vi "Process Records.vi"(4 "map from message info to indexes":T1, 5 "RT hardware channel data":T2[](array[typedef])=[{"channel #"=0, "channel handle"=0, "labels settings for RT"=[]}] {"labels settings for RT"."Label Timestamp Channel Data Reference" format="%.0x"; "labels settings for RT"."Word Initial Raw Value" format="%032.0f"; "labels settings for RT"."Label Disable/Trigger Channel Reference" format="%.0x"; "labels settings for RT"."parameter driver data"."Tx parameter refs" format="%.0x"; "labels settings for RT"."SDI" format="%02b"; "labels settings for RT"."label" format="%.0o"}, 6 "error in":errorcluster, 8 "map from message info to data word":T11(c390), 9 "parameter values in":dbl[](array[numeric])) -> (0 "error out":errorcluster, 3 "parameter values out":dbl[](array[numeric]))   [LabVIEW 2020, in "AIM ARINC 429 Engine.lvlib" / "Custom Device.lvlib"]
uses:
  Custom Device.lvlib
  ece6b673-d70a-4abd-8fc5-cd5ecd079ce2.vi
  <vilib>/NI VeriStand/Custom Device API/Data Reference.ctl
  <vilib>/NI VeriStand/Custom Device API/Custom Device API.lvlib
  <vilib>/NI VeriStand/Custom Device API/Custom Device Item Ref.ctl
  Shared/Label.ctl
  <vilib>/NI/NI VeriStand Encoding and Decoding/Encoding.ctl
  <vilib>/NI/NI VeriStand Encoding and Decoding/Encoding and Decoding.lvlib
  Shared/Parameter Definition.ctl
  Shared/RT Parameters.ctl
  Shared/Transfer Type.ctl
  Shared/RT Label Settings.ctl
  Shared/RT Hardware Channel Settings.ctl
  Shared/Map of Identifiers to Indexes.ctl
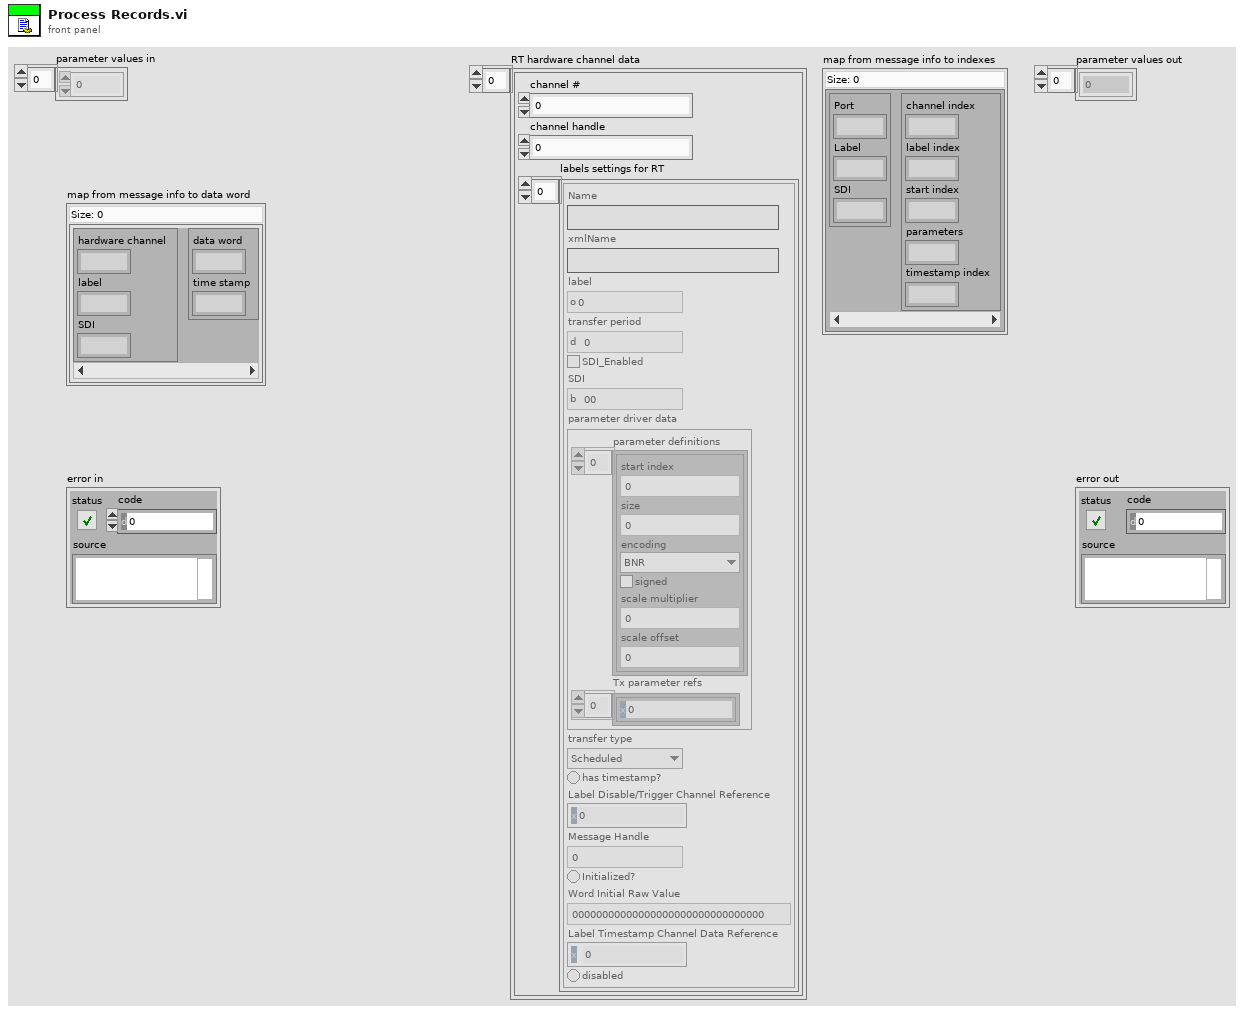
[diagram p1: front panel]
types:
  T1 = typedef "Map of Identifiers to Indexes.ctl" = map{cluster{"Port":u8, "Label":u8, "SDI":u8}, cluster{"channel index":i32, "label index":i32, "start index":i32, "parameters":i32, "timestamp index":i32}}
  T2 = typedef "RT Hardware Channel Settings.ctl" = cluster{"channel #":u16, "channel handle":u64, "labels settings for RT":T3[]}
  T3 = typedef "RT Label Settings.ctl" = cluster{"Name":string, "xmlName":string, "label":T4, "transfer period":u32, "SDI_Enabled":bool, "SDI":u8, "parameter driver data":T5, "transfer type":T9, "has timestamp?":bool, "Label Disable/Trigger Channel Reference":T8, "Message Handle":u64, "Initialized?":bool, "Word Initial Raw Value":u32, "Label Timestamp Channel Data Reference":T10, "disabled":bool}
  T4 = typedef "Label.ctl" = u8
  T5 = typedef "RT Parameters.ctl" = cluster{"parameter definitions":T6[], "Tx parameter refs":T8[]}
  T6 = typedef "Parameter Definition.ctl" = cluster{"start index":i32, "size":i32, "encoding":T7, "signed":bool, "scale multiplier":dbl, "scale offset":dbl}
  T7 = typedef "Encoding and Decoding.lvlib/Encoding.ctl" = enum16{"BNR", "BCD", "Discrete"}
  T8 = typedef "Custom Device API.lvlib/Custom Device Item Ref.ctl" = u64
  T9 = typedef "Transfer Type.ctl" = enum16{"Scheduled", "Acyclic", "Block", "Strobe"}
  T10 = typedef "Custom Device API.lvlib/Data Reference.ctl" = i32
  T11 = map{cluster{"hardware channel":u8, "label":u8, "SDI":u8}, cluster{"data word":u32, "time stamp":dbl}}
  T12 = cluster{"hardware channel":u8, "label":u8, "SDI":u8}
  T13 = cluster{"channel index":i32, "label index":i32, "start index":i32, "parameters":i32, "timestamp":i32}
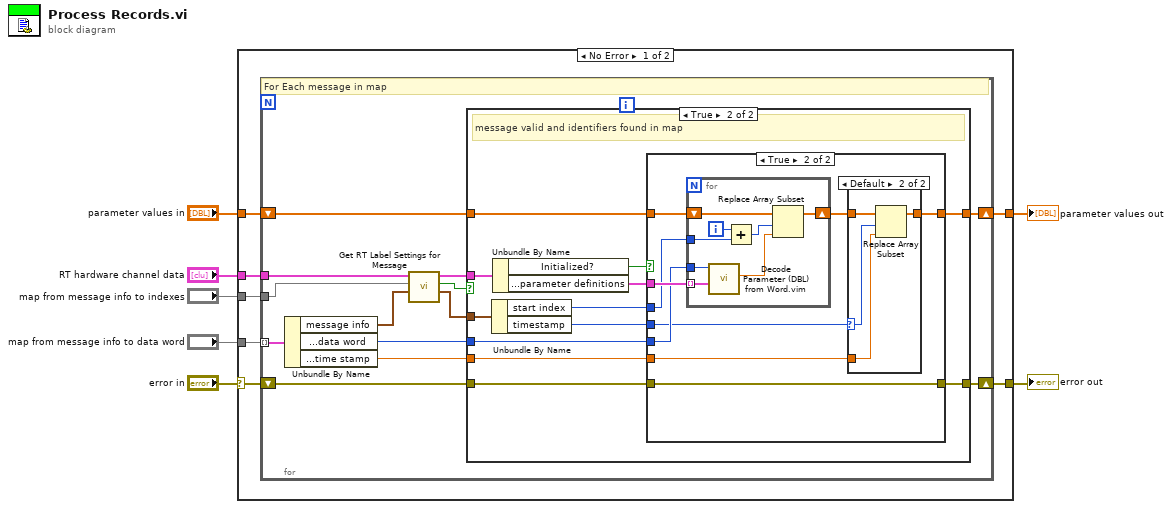
[diagram p0: block diagram]
diagram:
  n1 = case shown="No Error" "error in" {
    selector: "error in" -> [w12 w67]
    tunnel: "map from message info to data word" -> [w11 _]
    tunnel: [w14 w67] -> w6
    tunnel: "RT hardware channel data" -> [w13 _]
    tunnel: [w9 w66] -> w3
    tunnel: "parameter values in" -> [w10 w66]
    tunnel: "map from message info to indexes" -> [w8 _]
    frame No Error {
      n2 = for "Process each Record" {
        tunnel: w11 -> [w16] mode=indexing
        shift-right: [w27] -> w14
        shift-left: w12 -> [w26]
        tunnel: w13 -> [w23]
        shift-right: [w24] -> w9
        shift-left: w10 -> [w25]
        tunnel: w8 -> [w21]
        # "For Each message in map"
        n3 = Unbundle By Name(w16) -> ("message info"=w18:T12, "data word and time stamp.data word"=w17:u32, "data word and time stamp.time stamp"=w15:dbl)
        n4 = call "Get RT Label Settings for Message.vi"("message identifiers"=w18, "map"=w21, "RT hardware channel data"=w23) -> ("message indexes"=w19:T13, "valid and map exists"=w20:bool, "label settings for RT"=w22:T3)  [unwired: 6 in]
        n5 = case "Channel Found?" shown="True" w20 {
          tunnel: w26 -> [w29 w40]
          tunnel: [w29 w39] -> w27
          tunnel: w17 -> [_ w35]
          tunnel: [w28 w38] -> w24
          tunnel: w25 -> [w28 w36]
          tunnel: w22 -> [_ w34]
          tunnel: w19 -> [_ w33]
          tunnel: w15 -> [_ w31]
          frame False {
            # "message not valid or not found in map"
          }
          frame True {
            # "message valid and identifiers found in map"
            n6 = Unbundle By Name(w33) -> ("start index"=w32:i32, "timestamp"=w30:i32)
            n7 = Unbundle By Name(w34) -> ("Initialized?"=w37:bool, "parameter driver data.parameter definitions"=w41:T6[])
            n8 = case shown="True" w37 {
              tunnel: w41 -> [_ w51]
              tunnel: w35 -> [_ w50]
              tunnel: w40 -> [w43 w52]
              tunnel: [w43 w52] -> w39
              tunnel: [w42 w46] -> w38
              tunnel: w36 -> [w42 w49]
              tunnel: w32 -> [_ w48]
              tunnel: w31 -> [_ w44]
              tunnel: w30 -> [_ w47]
              frame False {
                # "This case will be called if users has Labels present on the channel but didn't list them in XML file with \"monitor=false\" in the list.\n\nRecords returned by Read function will have labels (not filtered by HW)."
              }
              frame True {
                n9 = for {
                  tunnel: w51 -> [w65] mode=indexing
                  tunnel: w50 -> [w64]
                  tunnel: w48 -> [w59]
                  shift-right: [w61] -> w45
                  shift-left: w49 -> [w63]
                  i -> [w60]
                  n10 = call "Decode Parameter (DBL) from Word.vim"("parameter definition"=w65, "32-bit word in"=w64) -> ("parameter value"=w62:dbl)  [unwired: 7 in, 2 out]
                  n11 = Add(x=w60, y=w59) -> (x+y=w58:i32)
                  n12 = Replace Array Subset(array=w63, new element=w62, index=w58) -> (w61:dbl[])
                }
                n13 = case shown="Default" w47 {
                  selector: w47 -> [_ w55]
                  tunnel: [w53 w56] -> w46
                  tunnel: w45 -> [w53 w57]
                  tunnel: w44 -> [_ w54]
                  frame ..-1 {
                  }
                  frame Default {
                    n14 = Replace Array Subset(array=w57, new element=w54, index=w55) -> (w56:dbl[])
                  }
                }
              }
            }
          }
        }
      }
    }
    frame Error {
    }
  }
  "error out" <- w6
  "parameter values out" <- w3
